vi "Show status data.vi"(8 "error in (no error)":errorcluster, 11 "Message":string) -> (0 "error out":errorcluster, 3 "Ctl Refnum":refnum<vi>)   [LabVIEW 2013]
panel:
  # "Information screen"
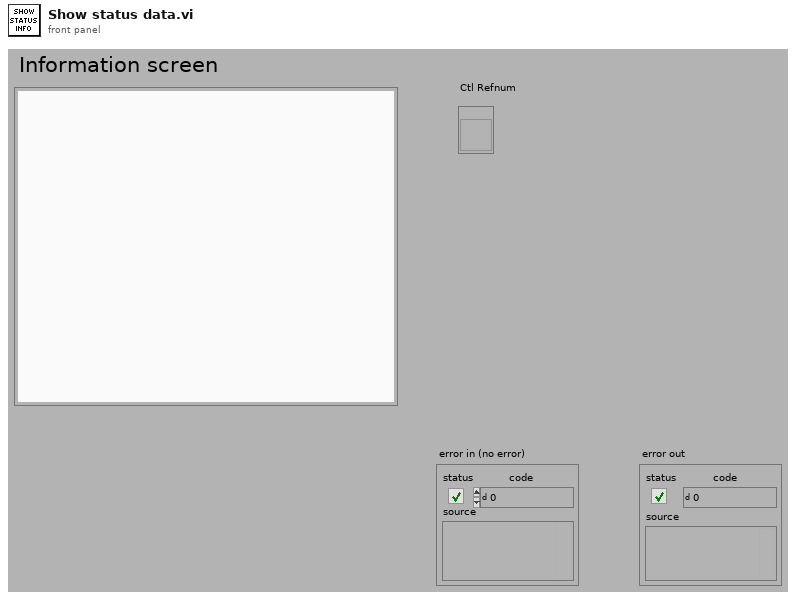
[diagram p1: front panel]
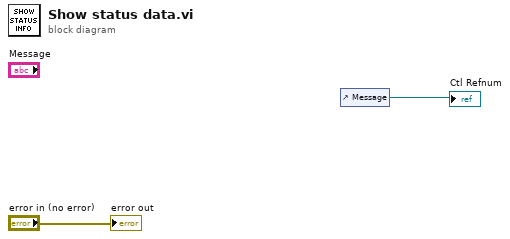
[diagram p0: block diagram]
diagram:
  n1 = control-ref of="Message"() -> (→"Ctl Refnum":refnum<vi>)
  "error out" <- "error in (no error)"
